vi "Command PRF.vi"(4 "VTxIndex":i8, 5 "Measurement Type":enum32{"Volt", "SA"}(radio), 6 "PID PRF":dbl=-95.93375, 7 "timeout (ms)":dbl=40000.0 format="%.2f", 8 "error in (no error)":errorcluster, 9 "Previous PRF":dbl, 10 "Voltage":dbl, 11 "TCP from Orchid in":refnum<k5>) -> (0 "error out":errorcluster, 2 "PRF":dbl)   [LabVIEW 2016]
doc: "This VI sets the Z system transmit parameters for an intensity measurement, reads them back, and checks for errors. It first gets the initial center element delay (TxpgDelayAperA) and the system frequencies using tcpSysTxFreqFromZ.vi. It then sets the elevation aperture (using SetZElevAper.vi), channel modulation, wavestyle, frequency, focus, number of transmit elements, number of cycles, voltage, and voltage channel, in that order. It reads back the settings (using tcpReadIntenSettingsZ.vi) and checks for errors. The final trigger delay and change in delay, in microseconds, are calculated from the initial and final values of TxpgDelayAperA using:\ndelay(us) = (TxpgDelayAperA + 178.0) / 160"
uses:
  TemperatureMeasure/Thermal_type.vi
panel:
  # "Program constants"
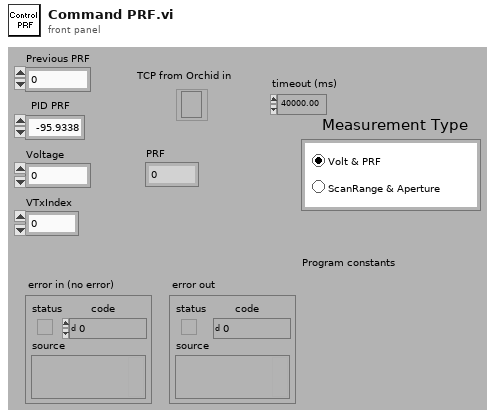
[diagram p1: front panel]
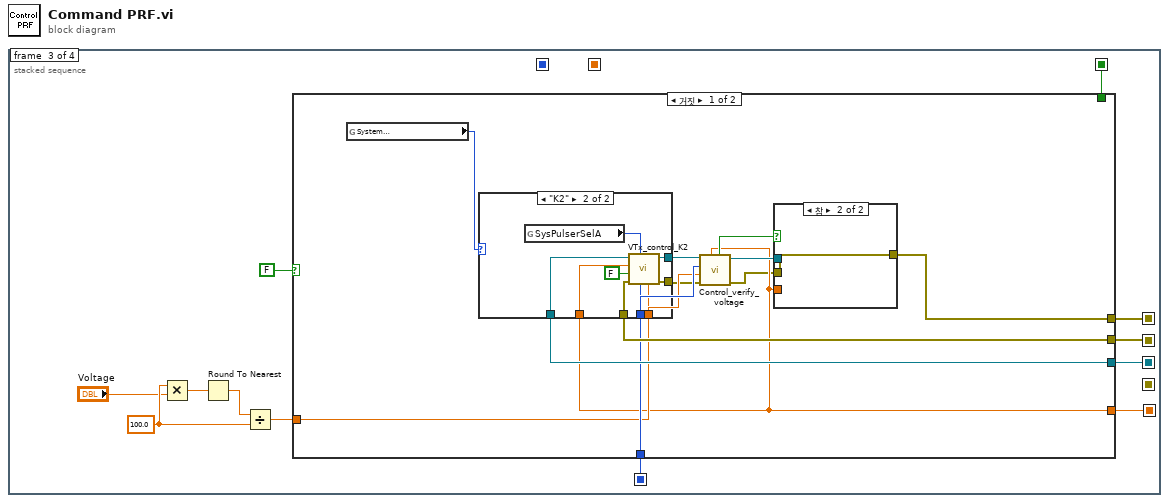
[diagram p0: block diagram]
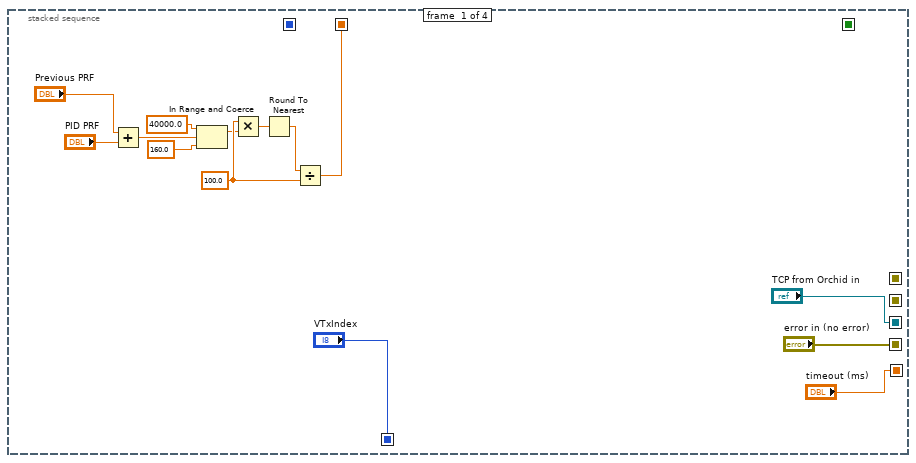
[diagram p2: hidden frame]
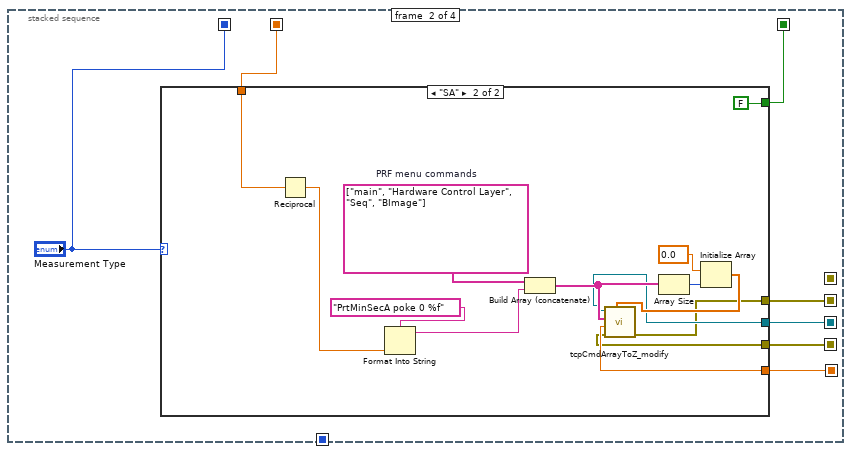
[diagram p3: hidden frame]
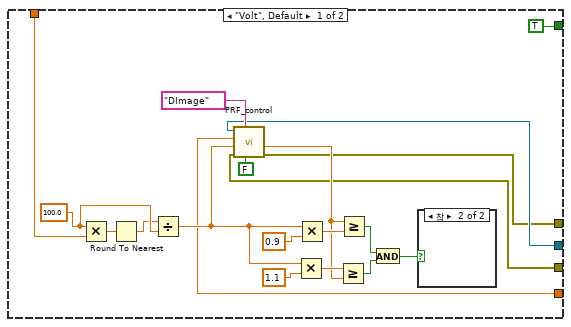
[diagram p4: hidden frame]
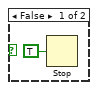
[diagram p5: hidden frame]
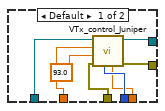
[diagram p6: hidden frame]
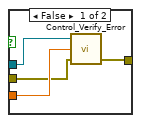
[diagram p7: hidden frame]
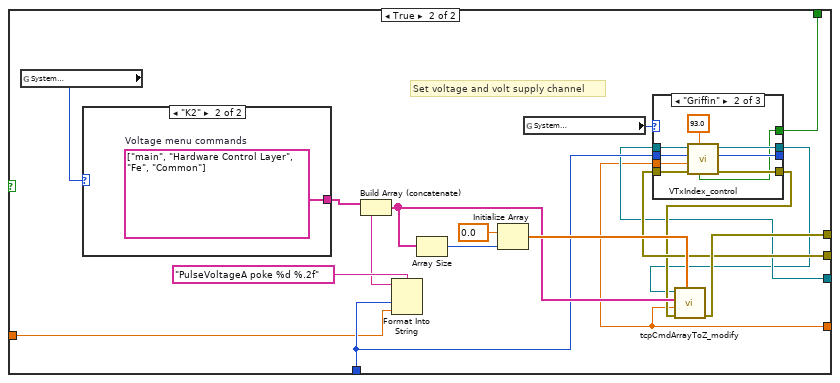
[diagram p8: hidden frame]
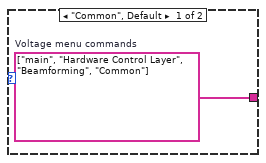
[diagram p9: hidden frame]
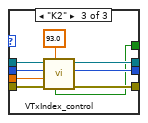
[diagram p11: hidden frame]
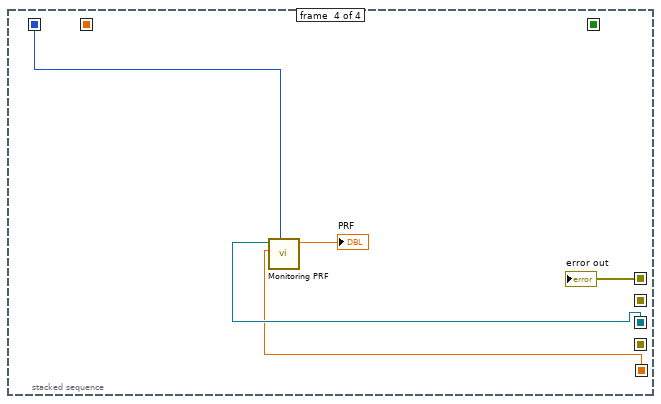
[diagram p12: hidden frame]
diagram:
  n1 = stacked-sequence {
    seq-local: ["TCP from Orchid in" _ _ _] -> [_ w19 w65 w147]
    seq-local: ["timeout (ms)" _ _ _] -> [_ w20 w64 w146]
    seq-local: ["error in (no error)" _ _ _] -> [_ w21 _ _]
    seq-local: [_ w18 _ _] -> [_ _ w67 _]
    seq-local: [w8 _ _ _] -> [_ w17 _ _]
    seq-local: [_ _ w68 _] -> [_ _ _ w148]
    seq-local: [_ "Measurement Type" _ _] -> [_ _ _ w144]
    seq-local: ["VTxIndex" _ _ _] -> [_ _ w66 _]
    seq-local: [_ w15 _ _] -> [_ _ w63 _]
    frame #0 {
      w10 = 100.0
      n2 = Add(x="Previous PRF", y="PID PRF") -> (x+y=w3:dbl)
      n3 = In Range and Coerce(upper limit=40000.0 ("y"), x=w3, lower limit=160.0 ("하위 리미트")) -> (coerced(x)=w2:dbl)  [unwired: 1 out]
      n4 = Multiply(x=w10, y=w2) -> (x*y=w11:dbl)
      n5 = Round To Nearest(number=w11) -> (nearest integer value=w9:dbl)
      n6 = Divide(x=w9, y=w10) -> (x/y=w8:dbl)
    }
    frame #1 {
      n7 = case shown="\"SA\"" "Measurement Type" {
        tunnel: w21 -> [w25 w46]
        tunnel: w20 -> [w26 w47]
        tunnel: w19 -> [w27 w48]
        tunnel: [w24 w45] -> w18
        tunnel: w17 -> [w23 w44]
        tunnel: [TRUE FALSE] -> w15
        frame "Volt", Default {
          w32 = 100.0
          n8 = Multiply(x=w32, y=w23) -> (x*y=w33:dbl)
          n9 = Round To Nearest(number=w33) -> (nearest integer value=w31:dbl)
          n10 = Divide(x=w31, y=w32) -> (x/y=w28:dbl)
          n11 = call "PRF_control.vi"("PRF_Event Down"=FALSE, "mode selection"="DImage", "error in (no error)"=w25, "Input PRF"=w28, "timeout (ms)"=w26, "TCP from Orchid in"=w27) -> ("error out"=w24:errorcluster, "PRF"=w30:dbl)  [unwired: 1 in, 1 out]
          n12 = Multiply(x=w28, y=1.1) -> (x*y=w38:dbl)
          n13 = Multiply(x=w28, y=0.9) -> (x*y=w34:dbl)
          n14 = Greater Or Equal?(x=w38, y=w30) -> (x >= y?=w37:bool)
          n15 = Greater Or Equal?(x=w30, y=w34) -> (x >= y?=w36:bool)
          n16 = And(x=w36, y=w37) -> (x .and. y?=w35:bool)
          n17 = case shown="참" w35 {
            frame False {
              n18 = Stop(stop? (T)=TRUE ("정지? (참)")) -> ()
            }
            frame True {
            }
          }
        }
        frame "SA" {
          w55 = string[] ["main", "Hardware Control Layer", "Seq", "BImage"]  # PRF menu commands
          n19 = Reciprocal(x=w44) -> (1/x=w49:dbl)
          n20 = Format Into String(format string="PrtMinSecA poke 0 %f", w49) -> (resulting string=w54:string)  [unwired: 2 in, 1 out]
          n21 = Build Array (concatenate)(w55, w54) -> (w51:string[])
          n22 = Array Size(array=w51) -> (size(s)=w53:i32)
          n23 = Initialize Array(0.0 ("element"), w53) -> (w50:dbl[])
          n24 = call "tcpCmdArrayToZ_modify.vi"("Delay (sec)"=w50, "error in (no error)"=w46, "Timeout (ms)"=w47, "Command array"=w51, "connection ID in"=w48) -> ("error out"=w45:errorcluster)  [unwired: 2 in, 4 out]
        }
      }
    }
    frame #2 {
      w60 = 100.0
      n25 = Multiply(x=w60, y="Voltage") -> (x*y=w59:dbl)
      n26 = Round To Nearest(number=w59) -> (nearest integer value=w61:dbl)
      n27 = Divide(x=w61, y=w60) -> (x/y=w57:dbl)
      n28 = case shown="거짓" FALSE {
        tunnel: [w70 w114] -> w68
        tunnel: w67 -> [w79 w112]
        tunnel: w66 -> [w77 w110]
        tunnel: w65 -> [w80 w109]
        tunnel: w64 -> [w72 w108]
        tunnel: w63 -> [_ w106]
        tunnel: w57 -> [w76 w103]
        frame False {
          n29 = global read "Thermal_type.vi" "System \nSelection"() -> (w69:enum32{"Common", "Frosk", "Griffin", "K2"})
          n30 = case shown="\"K2\"" w69 {
            tunnel: w80 -> [w88 w97]
            tunnel: w79 -> [w85 w96]
            tunnel: [w81 w93] -> w78
            tunnel: w77 -> [w84 w92]
            tunnel: w76 -> [w83 w91]
            tunnel: [w82 w90] -> w75
            tunnel: w72 -> [w87 w89]
            frame Default {
              n31 = call "VTx_control_Juniper.vi"("VTx_Voltage"=w83, "VTxIndex_In"=w84, "error in (no error)"=w85, "VTx1_voltage"=93.0, "Timeout (ms)"=w87, "connection ID in"=w88) -> ("error out"=w82:errorcluster, "connection ID out"=w81:refnum<k5>)  [unwired: 4 in]
            }
            frame "K2" {
              n32 = global read "Thermal_type.vi" "SysPulserSelA"() -> (w94:i16)
              n33 = call "VTx_control_K2.vi"("VTx_Voltage"=w91, "VTxIndex_In"=w92, "SystemPulerSelA"=w94, "error in (no error)"=w96, "CW/SCW"=FALSE, "Timeout (ms)"=w89, "connection ID in"=w97) -> ("error out"=w90:errorcluster, "connection ID out"=w93:refnum<k5>)  [unwired: 3 in]
            }
          }
          n34 = call "Control_verify_voltage.vi"("Timeout (ms)"=w72, "에러 입력(에러 없음)"=w75, "VTx_Voltage"=w76, "VTxIndex_In"=w77, "TCP 네트워크 연결 입력"=w78) -> ("에러 출력"=w71:errorcluster, "TCP 네트워크 연결 출력"=w73:refnum<k5>, "Verify_voltage"=w74:bool)  [unwired: 2 in, 2 out]
          n35 = case shown="참" w74 {
            tunnel: w73 -> [w101 _]
            tunnel: w72 -> [w100 _]
            tunnel: w71 -> [w99 w102]
            tunnel: [w98 w102] -> w70
            frame False {
              n36 = call "Control_Verify_Error.vi"("에러 입력(에러 없음)"=w99, "timeout (ms)"=w100, "TCP 네트워크 연결 입력"=w101) -> ("에러 출력"=w98:errorcluster)  [unwired: 2 in]
            }
            frame True {
            }
          }
        }
        frame True {
          # "Set voltage and volt supply channel"
          n37 = global read "Thermal_type.vi" "System \nSelection"() -> (w105:enum32{"Common", "Frosk", "Griffin", "K2"})
          n38 = case shown="\"K2\"" w105 {
            tunnel: [w121 w122] -> w104
            frame "Common", Default {
              w121 = string[] ["main", "Hardware Control Layer", "Beamforming", "Common"]  # Voltage menu commands
            }
            frame "K2" {
              w122 = string[] ["main", "Hardware Control Layer", "Fe", "Common"]  # Voltage menu commands
            }
          }
          n39 = Format Into String(format string="PulseVoltageA poke %d %.2f" ("Format String"), w110, w103) -> (resulting string=w119:string)  [unwired: 2 in, 1 out]
          n40 = Build Array (concatenate)(w104, w119) -> (w115:string[])
          n41 = Array Size(array=w115) -> (size(s)=w118:i32)
          n42 = Initialize Array(0.0 ("element"), w118) -> (w116:dbl[])
          n43 = global read "Thermal_type.vi" "System \nSelection"() -> (w113:enum32{"Common", "Frosk", "Griffin", "K2"})
          n44 = case shown="\"Griffin\"" w113 {
            tunnel: w109 -> [w125 w134 w143]
            tunnel: w110 -> [w124 w132 w141]
            tunnel: w108 -> [_ w131 w140]
            tunnel: [w125 w130 w139] -> w107
            tunnel: [w124 w129 w138] -> _
            tunnel: w112 -> [w123 w128 w137]
            tunnel: [w123 w127 w136] -> w111
            tunnel: w106 -> [_ w126 w135]
            frame "Common", "Frosk", Default {
            }
            frame "Griffin" {
              n45 = call "VTxIndex_control.vi"("Is_D_mode"=w126, "VTx1_volt"=93.0, "error in (no error)"=w128, "Timeout (ms)"=w131, "VTxIndex_In"=w132, "connection ID in"=w134) -> ("error out"=w127:errorcluster, "VTxIndex_Out"=w129:i8, "connection ID out"=w130:refnum<k5>)  [unwired: 3 in]
            }
            frame "K2" {
              n46 = call "VTxIndex_control.vi"("Is_D_mode"=w135, "VTx1_volt"=93.0, "error in (no error)"=w137, "Timeout (ms)"=w140, "VTxIndex_In"=w141, "connection ID in"=w143) -> ("error out"=w136:errorcluster, "VTxIndex_Out"=w138:i8, "connection ID out"=w139:refnum<k5>)  [unwired: 3 in]
            }
          }
          n47 = call "tcpCmdArrayToZ_modify.vi"("Delay (sec)"=w116, "error in (no error)"=w111, "Timeout (ms)"=w108, "Command array"=w115, "connection ID in"=w107) -> ("error out"=w114:errorcluster)  [unwired: 2 in, 4 out]
        }
      }
    }
    frame #3 {
      n48 = call "Monitoring PRF.vi"("Measurement Type"=w144, "timeout (ms)"=w146, "TCP from Orchid in"=w147) -> ("PRF"=→"PRF":dbl)  [unwired: 6 in, 1 out]
      "error out" <- w148
    }
  }
